vi "Reset Abort.vi"(8 "error in (no error)":errorcluster, 11 "DataProcessor in":refnum<class "DataProcessor.lvclass">) -> (0 "error out":errorcluster, 3 "DataProcessor out":refnum<class "DataProcessor.lvclass">)   [LabVIEW 2020, in "Volatus.lvlib" / "DataProcessor.lvclass"]
uses:
  DataProcessor.lvclass
  DataProcessor.lvclass/DataProcessor.ctl
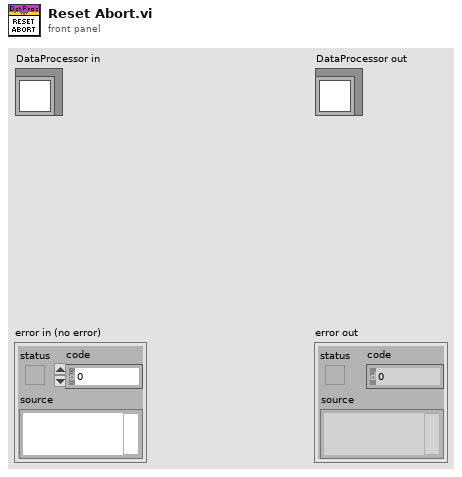
[diagram p1: front panel]
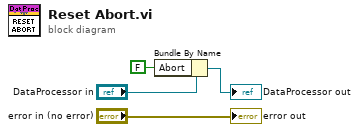
[diagram p0: block diagram]
diagram:
  n1 = Bundle By Name(cluster="DataProcessor in", "Abort"=FALSE) -> (→"DataProcessor out":refnum<class "DataProcessor.lvclass">)
  "error out" <- "error in (no error)"
